vi "Projectile.vi"() -> ()   [LabVIEW 2013]
panel:
  out "XY Graph":cluster{"theta":i32[], "R":dbl[]}(graph)
  in  "Launch Height (m)":dbl
  in  "Launch Speed (m/s)":dbl
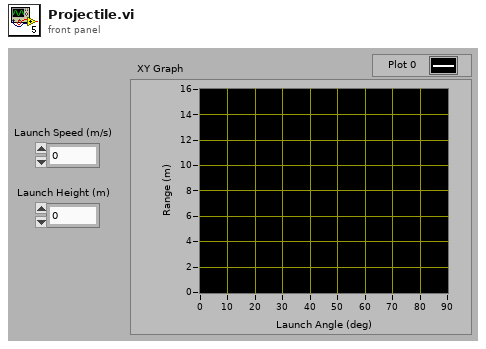
[diagram p1: front panel]
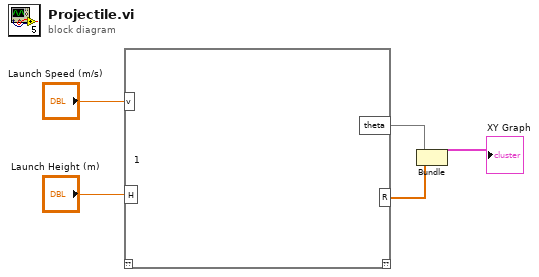
[diagram p0: block diagram]
diagram:
  n1 = mathscript code="1"("v"="Launch Speed (m/s)", "H"="Launch Height (m)") -> ("theta"=w5, "R"=w4:dbl[])  [unwired: 1 in, 1 out]
  n2 = Bundle("theta"=w5, "R"=w4) -> (→"XY Graph":cluster{"theta":void, "R":dbl[]})  [unwired: 1 in]
